vi "Simulate 3 Phase Power.vi"(6 "sampling info":cluster{"Fs":dbl, "#s":dbl}={"Fs"=1000.0, "#s"=1000.0} {"Fs" format="%.2p"}, 7 "Reset":bool, 8 "error in":errorcluster, 9 "Harmonics Array":T2(array[cluster]), 10 "Fundamental Array":cluster{"level (%)":dbl, "phase (°)":dbl}[](array[cluster]), 11 "Frequency and Amplitude":T1={"frequency (Hz)"=60.0, "voltage (V) RMS"=1.0, "current (A) RMS"=5.0} {"current (A) RMS" scale=0.0..50.0; "voltage (V) RMS" scale=0.0..300.0; "frequency (Hz)" scale=40.0..60.0}) -> (0 "error out":errorcluster, 3 "Wfm data":waveform(dbl)[](array[waveform]))   [LabVIEW 2024]
uses:
  <vilib>/measure/NI_MABase.lvlib
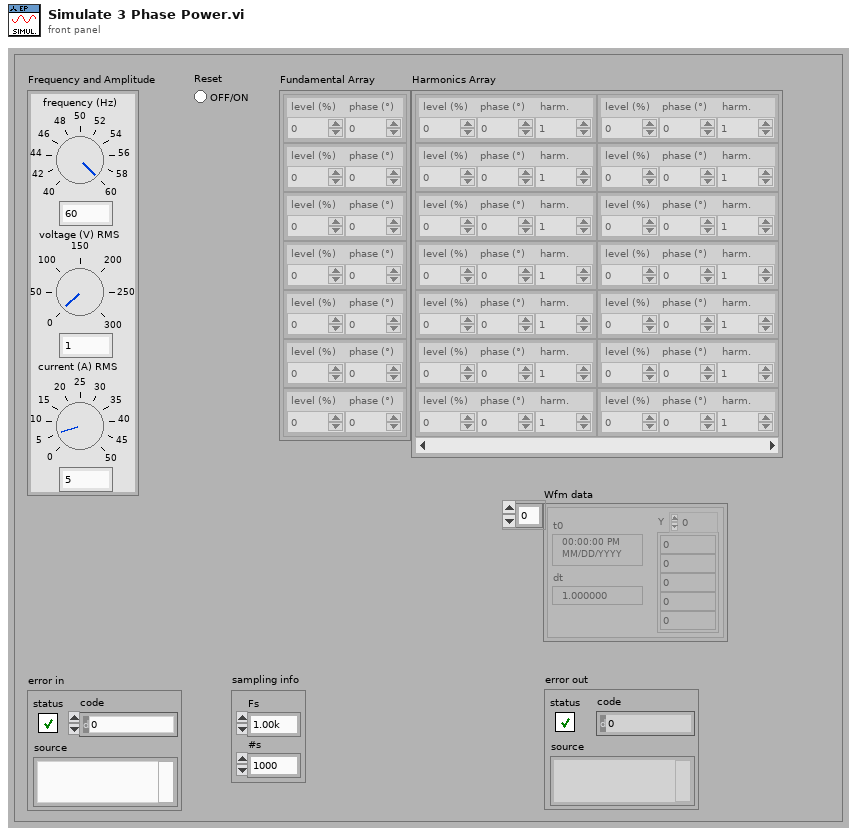
[diagram p1: front panel]
types:
  T1 = cluster{"frequency (Hz)":sgl, "voltage (V) RMS":dbl, "current (A) RMS":dbl}
  T2 = cluster{"level (%)":dbl, "phase (°)":dbl, "harm.":dbl}[][]
  T3 = cluster{"level (%)":dbl, "phase (°)":dbl, "harm.":dbl}
  T4 = enum16{"Sine Wave", "Triangle Wave", "Square Wave", "Sawtooth Wave"}
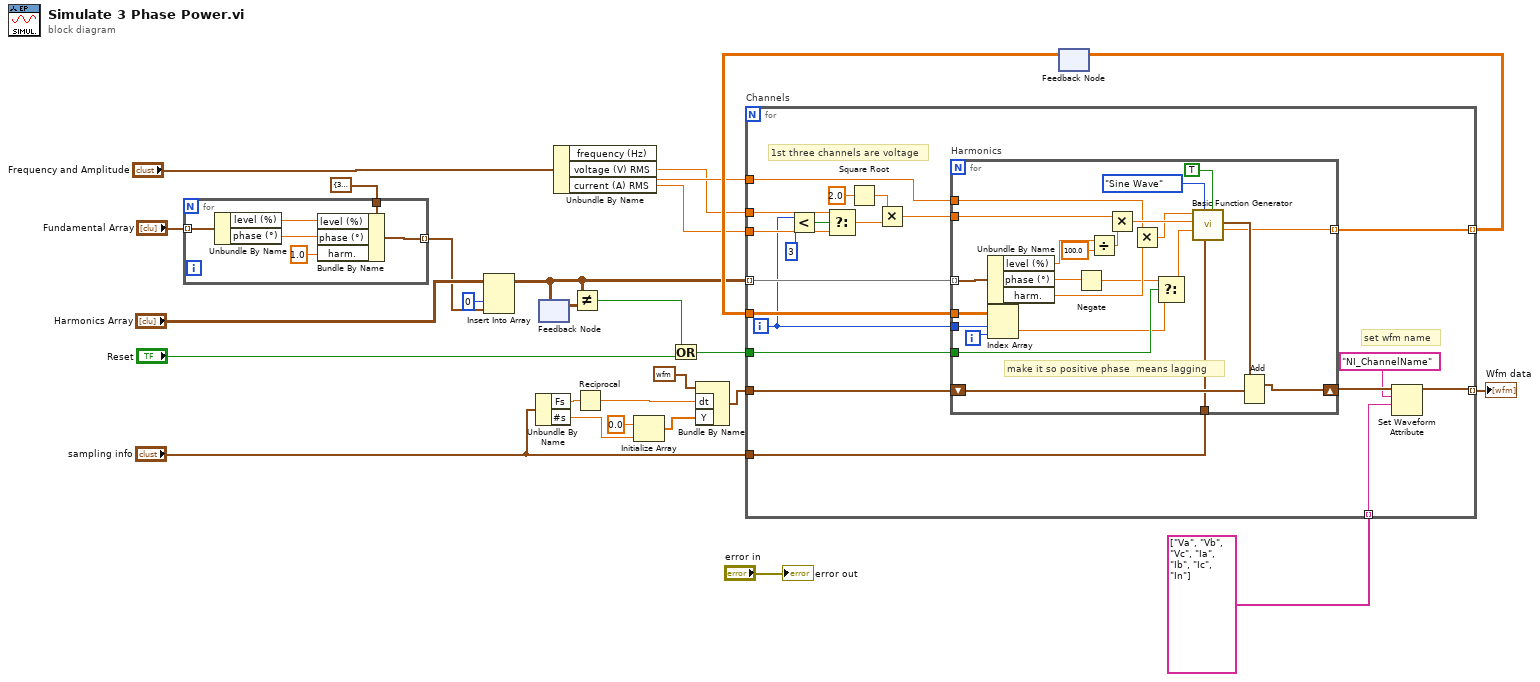
[diagram p0: block diagram]
diagram:
  n1 = for {
    tunnel: T3 {"level (%)"=3.0, "phase (°)"=0.0, "harm."=3.0} ("Harmonic") -> [w33]
    tunnel: "Fundamental Array" -> [w30] mode=indexing
    tunnel: [w32] -> w5 mode=indexing
    n2 = Unbundle By Name(w30) -> ("level (%)"=w29:dbl, "phase (°)"=w28:dbl)
    n3 = Bundle By Name(cluster=w33, "level (%)"=w29, "phase (°)"=w28, "harm."=1.0) -> (w32:T3)
  }
  n4 = Insert Into Array(array="Harmonics Array", index (col)=0 ("disabled index (col)"), new element=w5) -> (w3:T2)  [unwired: 1 in]
  n5 = Unbundle By Name("sampling info") -> ("Fs"=w16:dbl, "#s"=w14:dbl)
  n6 = feedback-in #1(w3) -> ()
  n7 = feedback #1() -> (w25:T2)  [unwired: 1 in]
  n8 = Unbundle By Name("Frequency and Amplitude") -> ("frequency (Hz)"=w11:sgl, "voltage (V) RMS"=w10:dbl, "current (A) RMS"=w9:dbl)
  n9 = Not Equal?(x=w3, y=w25) -> (x != y?=w24:bool)
  n10 = Reciprocal(x=w16) -> (1/x=w15:dbl)
  n11 = Initialize Array(0.0 ("element"), w14) -> (w13:dbl[])
  n12 = Or(x=w24, y="Reset") -> (x .or. y?=w26:bool)
  n13 = Bundle By Name(cluster=waveform(dbl) {"t0"=timestamp(0 s since 1904-01-01), "dt"=1.0, "Y"=[]} ("signal out"), "dt"=w15, "Y"=w13) -> (w17:waveform(dbl))
  n14 = feedback #2() -> (w22:dbl[][])  [unwired: 1 in]
  n15 = for "Channels" {
    tunnel: [w53] -> w23 mode=indexing
    tunnel: w10 -> [w52]
    tunnel: w9 -> [w51]
    tunnel: w3 -> [w47] mode=indexing
    tunnel: w22 -> [w46]
    tunnel: w26 -> [w45]
    tunnel: [w36] -> w20 mode=indexing
    tunnel: "sampling info" -> [w42]
    tunnel: w11 -> [w41]
    tunnel: w17 -> [w40]
    tunnel: string[] ["Va", "Vb", "Vc", "Ia", "Ib", "Ic", "In"] -> [w34] mode=indexing
    i -> [w39]
    # "set wfm name"
    # "1st three channels are voltage"
    n16 = Less?(x=w39, y=3) -> (x < y?=w44:bool)
    n17 = Select(t=w52, s=w44, f=w51) -> (s? t:f=w43:dbl)
    n18 = Square Root(x=2.0) -> (sqrt(x)=w49:dbl)
    n19 = Multiply(x=w49, y=w43) -> (x*y=w48:dbl)
    n20 = for "Harmonics" {
      shift-right: [w56] -> w37
      shift-left: w40 -> [w77]
      tunnel: [w62] -> w53 mode=indexing
      tunnel: w48 -> [w72]
      tunnel: w47 -> [w76] mode=indexing
      tunnel: w46 -> [w67]
      tunnel: w45 -> [w70]
      tunnel: w39 -> [w69]
      tunnel: w42 -> [w59]
      tunnel: w41 -> [w58]
      i -> [w68]
      # "make it so positive phase  means lagging"
      n21 = Unbundle By Name(w76) -> ("level (%)"=w75:dbl, "phase (°)"=w55:dbl, "harm."=w71:dbl)
      n22 = Index Array(array=w67, index (row)=w69, index (col)=w68) -> (element=w66:dbl)
      n23 = Negate(x=w55) -> (-x=w54:dbl)
      n24 = Divide(x=w75, y=100.0) -> (x/y=w73:dbl)
      n25 = Multiply(x=w72, y=w73) -> (x*y=w64:dbl)
      n26 = Multiply(x=w58, y=w71) -> (x*y=w57:dbl)
      n27 = Select(t=w54, s=w70, f=w66) -> (s? t:f=w61:dbl)
      n28 = call <vilib>:"Basic Function Generator.vi"("reset signal"=TRUE ("reset phase"), "sampling info"=w59, "signal type"=T4."Sine Wave", "phase"=w61, "amplitude"=w64, "frequency"=w57) -> ("phase out"=w62:dbl, "signal out"=w63:waveform(dbl))  [unwired: 3 in, 1 out]
      n29 = Add(1:w77, 2:w63) -> (0:w56:waveform(dbl))  [unwired: 1 in, 1 out]
    }
    n30 = Set Waveform Attribute(5:w34, 6:"NI_ChannelName" ("name"), 7:w37) -> (3:w36:waveform(dbl))  [unwired: 1 in, 2 out]
  }
  "Wfm data" <- w20
  n31 = feedback-in #2(w23) -> ()
  "error out" <- "error in"
